vi "DisplayResult.vi"(9 "Result Input":dbl, 10 "Y":dbl, 11 "X":dbl) -> ()   [LabVIEW 2014]
panel:
  out "Result is Currently:":dbl
  in  "OK Button":bool
  out "X is Currently:":dbl
  out "Y is Currently:":dbl
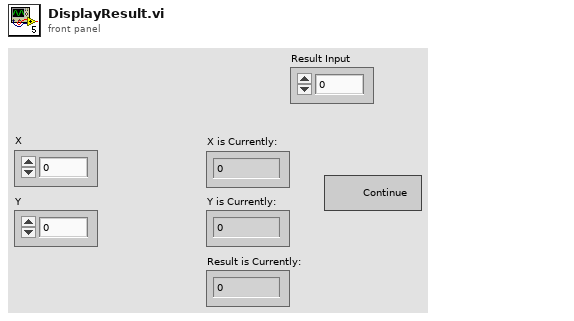
[diagram p1: front panel]
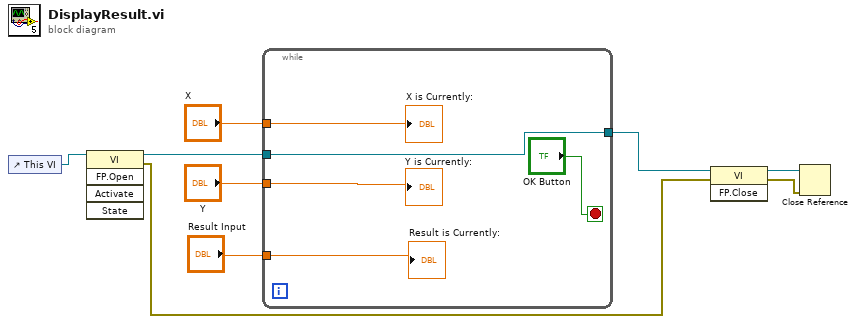
[diagram p0: block diagram]
diagram:
  n1 = control-ref of="This VI"() -> (w6:refnum<vi>)
  n2 = invoke class="VI" method="FP.Open"(reference=w6) -> (reference out=w3:refnum<vi>, error out=w1:errorcluster)  [unwired: 4 in, 3 out]
  n3 = while {
    tunnel: "Result Input" -> [w13]
    tunnel: "Y" -> [w12]
    tunnel: "X" -> [w11]
    tunnel: w3 -> [w10]
    tunnel: [w10] -> w2
    stop <- "OK Button" stop-if-true
    "Y is Currently:" <- w12
    "X is Currently:" <- w11
    "Result is Currently:" <- w13
  }
  n4 = invoke class="VI" method="FP.Close"(reference=w2, error in=w1) -> (reference out=w5:refnum<vi>, error out=w4:errorcluster)  [unwired: 1 in, 1 out]
  n5 = Close Reference(reference=w5, error in (no error)=w4) -> ()  [unwired: 1 out]
